vi "PH_Cam_BaseClass.Remove Image.vi"(0 "i ref in":refnum<vi>, 5 "error in":errorcluster) -> (14 "i ref out":refnum<vi>, 19 "error out":errorcluster)   [LabVIEW 2014, in "PH_Cam_BaseClass.lvlib"]
doc: "This Vi writes the current image position to the hard disk."
uses:
  PH_Cam_BaseClass.lvlib
  <vilib>/Utility/xml.llb/Write to XML File(string).vi
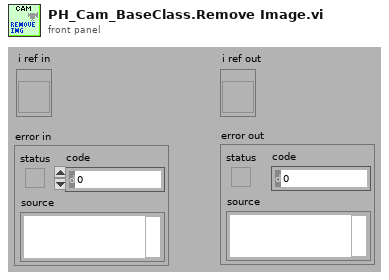
[diagram p1: front panel]
types:
  T1 = typedef "PH_Cam_BaseClass.lvlib/PH_Cam_BaseClass.i attribute.ctl" = cluster{"Gui Refs":T2, "Cam":cluster{"Source Notifier":refnum<notifier>, "Error":errorcluster, "Camera ID":string}, "Images":cluster{"Cam":T3, "Operation":T3, "PSDB":T3}, "Window Image":cluster{"Indicate Image":bool, "Window No.":i32, "Scale Facor":dbl, "Center Cross":bool, "Subtract Backgr":bool, "CoG":bool, "Color Palette":cluster{"Red":u8, "Green":u8, "Blue":u8}[], "Image On":bool}, "Default Prdc Int":i32, "Performance":cluster{"on":bool, "Timestamp Last Frame":i32}, "Histogram":cluster{"on":bool, "Mapping":bool}, "Save Image":cluster{"Save":bool, "File refnum":refnum<file>}, "Setting Service ID":i32, "Screen":cluster{"x-resolution":i16, "y-resolution":i16}, "On":bool, "Constructor finished":bool, "configured":bool}
  T2 = typedef "PH_Cam_BaseClass.lvlib/PH_Cam_BaseClass.GUI Refs.ctl" = cluster{"Frame Rate":refnum<vi>, "Get Frame Rate":refnum<vi>, "Show Image":refnum<vi>, "Get Histogram":refnum<vi>, "Mapping":refnum<vi>, "Histogram":refnum<vi>, "Center Cross":refnum<vi>, "Center of Gravity":refnum<vi>, "Scale Factor [%]":refnum<vi>, "Save Image":refnum<vi>, "Palette":refnum<vi>, "Subtract Background":refnum<vi>, "Cam Error":refnum<vi>, "On":refnum<vi>, "Cam List":refnum<vi>}
  T3 = typedef "IMAQ Image.ctl" = refnum<image>
  T4 = enum16{"open", "replace", "create", "open or create", "replace or create", "replace or create with confirmation"}
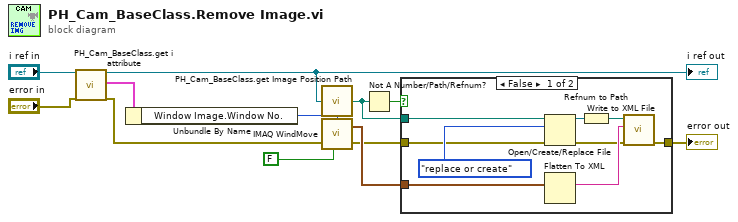
[diagram p0: block diagram]
diagram:
  n1 = call "PH_Cam_BaseClass.get i attribute.vi"("i ref in"="i ref in", "error in (no error)"="error in") -> ("i ref out"=w1:refnum<vi>, "i attribute"=w9:T1, "error out"=w11:errorcluster)  [unwired: 15 in]
  "i ref out" <- w1
  n2 = Unbundle By Name(w9) -> ("Window Image.Window No."=w7:i32)
  n3 = call "PH_Cam_BaseClass.get Image Position Path.vi"("i ref in"=w1) -> ("Image GUI Postion Path"=w2:path)
  n4 = call "IMAQ WindMove"("Window Number (0...15)"=w7, "Get/Set Status? (Set)"=FALSE, "error in (no error)"=w11) -> ("Coordinates (screen)"=w4:cluster{"X Position":i32, "Y Position":i32}, "error out"=w3:errorcluster)  [unwired: 2 in]
  n5 = Not A Number/Path/Refnum?(number/path/refnum=w2) -> (NaN/Path/Refnum?=w5:bool)
  n6 = case shown="False" w5 {
    tunnel: w4 -> [w20 _]
    tunnel: w2 -> [w19 _]
    tunnel: w3 -> [w14 w22]
    tunnel: [w17 w22] -> w8
    frame False {
      n7 = Open/Create/Replace File(file path (use dialog)=w19, error in=w14, operation (0:open)=T4."replace or create") -> (refnum out=w15:refnum<file>, error out=w13:errorcluster)  [unwired: 3 in, 1 out]
      n8 = Flatten To XML(anything=w20) -> (xml string=w21:string)
      n9 = Refnum to Path(1:w15) -> (0:w16:path)
      n10 = call-poly <vilib>:"Write to XML File.vi"("error in (no error)"=w13, "XML Input"=w21, "XML File Path"=w16) -> ("error out"=w17:errorcluster)  [unwired: 6 in, 2 out]
    }
    frame True {
    }
  }
  "error out" <- w8
